vi "AndorCheck.vi"(2 "error in":errorcluster, 3 "Input":i32) -> (0 "error out":errorcluster, 1 "Status":bool)   [LabVIEW 2014]
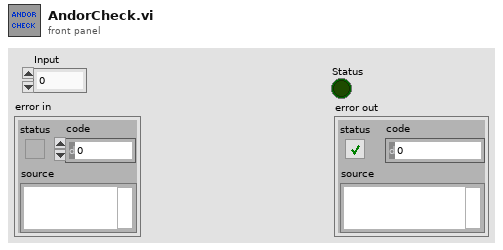
[diagram p1: front panel]
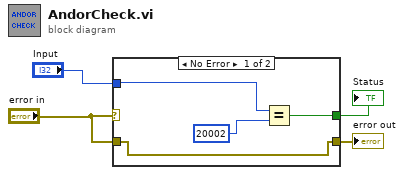
[diagram p0: block diagram]
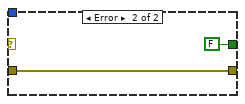
[diagram p2: hidden frame]
diagram:
  n1 = case shown="No Error" "error in" {
    tunnel: [w8 FALSE] -> w2
    tunnel: "error in" -> [w7 w10]
    tunnel: [w7 w10] -> w3
    tunnel: "Input" -> [w5 _]
    frame No Error {
      n2 = Equal?(x=w5, y=20002) -> (x = y?=w8:bool)
    }
    frame Error {
    }
  }
  "error out" <- w3
  "Status" <- w2
